vi "IndexVelocity_Read.vi"(0 "Axis In":T2, 5 "Index (0)":T1) -> (4 "Axis Out":T2, 6 "Index (duplicate)":T1, 8 "Velocity":dbl)   [LabVIEW 2009]
uses:
  typedefs/Ultra3000/Cmds.ctl
  typedefs/Ultra3000/Func.ctl
  globals/AxisSpace.vi
  typedefs/Ultra3000/Index_Numeric.ctl
  typedefs/AxisSelect_Enum.ctl
panel:
  out "error out":errorcluster
  in  "error in (no error)":errorcluster
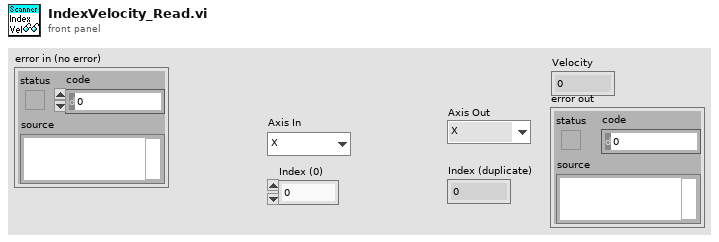
[diagram p1: front panel]
types:
  T1 = typedef "Index_Numeric.ctl" = u8
  T2 = typedef "AxisSelect_Enum.ctl" = enum16{"X", "Y", "Z", "Axis Space"}
  T3 = typedef "Func.ctl" = u16
  T4 = typedef "Cmds.ctl" = u16
  T5 = typedef "AxisSpaceCfg.ctl" = T6[]
  T6 = typedef "AxisCfg.ctl" = cluster{"Addr":u8, "Conv Factor":dbl, "Positive Limit":dbl, "Negative Limit":dbl}
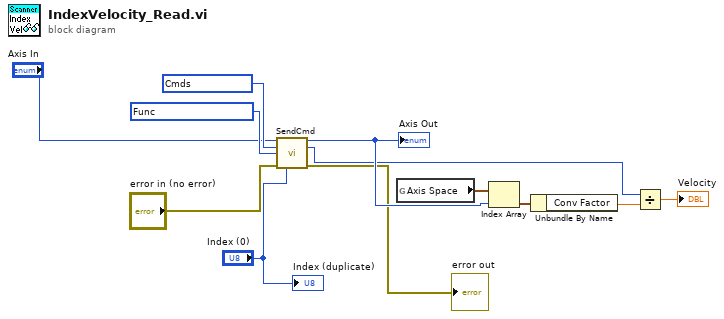
[diagram p0: block diagram]
diagram:
  w11 = T3 ? items=["Read Working Value", "Write Working Value", "Read Non-Volatile Value", "Write Non-Volatile and Woring Value", "Copy Non-Volatile Value to Working Value", "Copy Working Value to Non-Volatile Value", "Read Default Value", "Copy Default Value to Non-Volatile and Working Values", "Read Min Value", "Read Max Value", "Read Array Index Min", "Read Array Index Max"] ("Function")
  w12 = T4 ? items=["Position Command", "Run Status", "Fault Status", "Position Error", "Auto-Start Homing", "Start Homing", "Homing Type", "Motor Position", "Velocity Motor", "Power-Up Status", "Drive Name", "Position Window Size", "Position Window Time", "Zero Speed Limit", "Speed Window Size", "Up to Speed Limit", "Forward Current Limit", "Reverse Current Limit", "Override Mode", "Operation Mode", "Host Control Mode", "Reset Drive", "Drive Enable", "Setpoint Current", "Setpoint Velocity", "Setpoint Acceleration", "Reset Faults", "Position Comparator", "Postition Comparator Polarity", "Position Rollover Enable", "Baud Rate", "Frame Format", "Drive Address", "Broadcast Address", "Auto-start Indexing", "Start Index", "Host Index", "Index Type", "Index Dist/Pos", "Index Reg Dist", "Index Velocity", "Index Acceleration", "Index Deceleration", "Index Dwell", "Index Count", "Index Termination", "Index Pointer", "Index Abort Deceleration", "Positive Soft Pos Limit", "Define Home", "Negative Soft Pos Limit"] ("Command")
  n1 = call "SendCmd.vi"("Axis In"="Axis In", "Command"=w12, "Function"=w11, "error in (no error)"="error in (no error)", "Index (0)"="Index (0)") -> ("Axis Out"=w6:T2, "Data"=w4:i32, "error out"=→"error out":errorcluster)  [unwired: 7 in, 1 out]
  "Axis Out" <- w6
  n2 = global read "AxisSpace.vi" "Axis Space"() -> (w9:T5)
  n3 = Index Array(array=w9, index=w6) -> (element=w7:T6)
  n4 = Unbundle By Name(w7) -> ("Conv Factor"=w5:dbl)
  n5 = Divide(x=w4, y=w5) -> (x/y=→"Velocity":dbl)
  "Index (duplicate)" <- "Index (0)"
